vi "1.vi"() -> ()   [LabVIEW 2017]
panel:
  out "最大心率":dbl
  in  "年龄":dbl
  in  "年龄":enum16{"男", "女"}(ring)
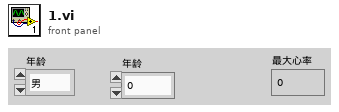
[diagram p1: front panel]
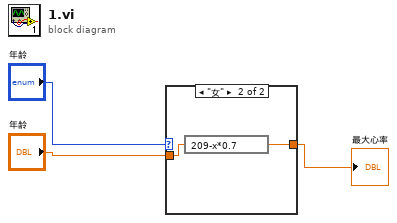
[diagram p0: block diagram]
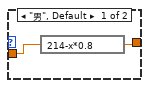
[diagram p2: hidden frame]
diagram:
  n1 = case shown="\"女\"" "年龄" {
    tunnel: [w5 w7] -> w1
    tunnel: "年龄" -> [w4 w6]
    frame "男", Default {
      n2 = expression code="214-x*0.8"(w4) -> (w5:dbl)
    }
    frame "女" {
      n3 = expression code="209-x*0.7"(w6) -> (w7:dbl)
    }
  }
  "最大心率" <- w1
